vi "client.vi"() -> ()   [LabVIEW 2019]
uses:
  Generated_client/RPC Messages/Greeter_req.ctl
  Generated_client/RPC Messages/Greeter_req_req_oneof/Greeter_req_req_oneof.lvclass
  Generated_client/RPC Messages/Greeter_req_req_oneof/Greeter_req_req_oneof.lvclass/Greeter_req_req_oneof.ctl
  Generated_client/RPC Messages/Greeter_res_res_oneof/Greeter_res_res_oneof.lvclass/Greeter_res_res_oneof.ctl
  Generated_client/Generated_client.lvlib
  Generated_client/RPC Messages/Greeter_res_res_oneof/Greeter_res_res_oneof.lvclass
panel:
  out "res_price":sgl format="%.2f"
  out "res_flag":bool
  out "res_num":i32
  out "res_name":string
  out "res_latitude":i32
  in  "req_latitude":i32=1011
  in  "req_price":sgl=123.0
  in  "flag":bool
  in  "req_num":i32=12
  in  "req_name":string="Dan"
  in  "req_oneof":u16(ring) items=["req_name", "req_num", "flag", "price"]
  out "error out":errorcluster
  in  "error in":errorcluster
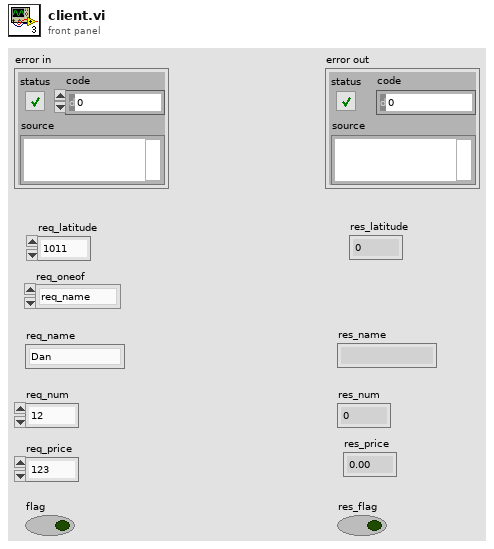
[diagram p1: front panel]
types:
  T1 = typedef "Generated_client.lvlib/Greeter_req.ctl" = cluster{"req_latitude":i32, "Greeter_req_req_oneof":refnum<class "Greeter_req_req_oneof.lvclass">}
  T2 = typedef "grpc-lvsupport-release.lvlib/grpcId.ctl" = u64
  T3 = typedef "Generated_client.lvlib/Greeter_res.ctl" = cluster{"res_latitude":i32, "Greeter_res_res_oneof":refnum<class "Greeter_res_res_oneof.lvclass">}
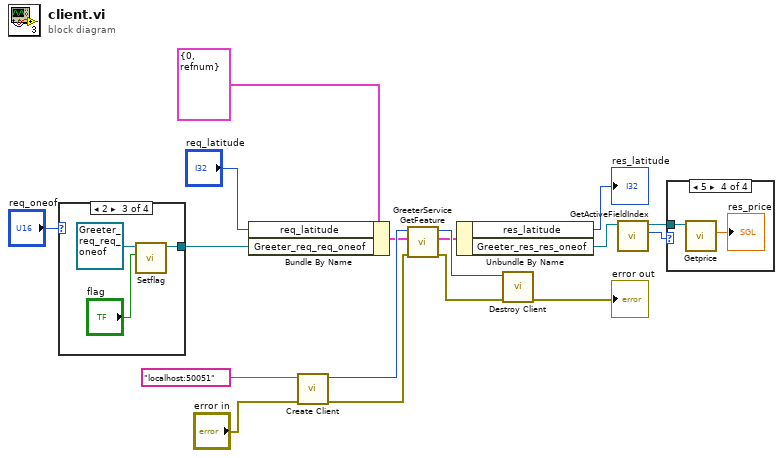
[diagram p0: block diagram]
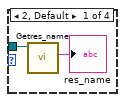
[diagram p2: hidden frame]
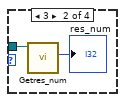
[diagram p3: hidden frame]
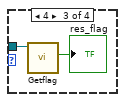
[diagram p4: hidden frame]
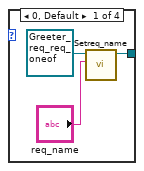
[diagram p5: hidden frame]
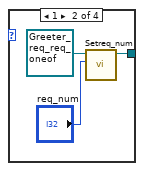
[diagram p6: hidden frame]
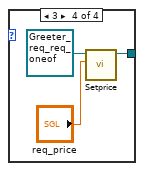
[diagram p7: hidden frame]
diagram:
  n1 = case shown="2" "req_oneof" {
    tunnel: [w18 w21 w26 w27] -> w7
    frame 0, Default {
      n2 = call "Setreq_name.vi"("Set_Val"="req_name", "OneOfTemplate in"=refnum<class "Greeter_req_req_oneof.lvclass"> refnum) -> ("OneOfTemplate out"=w18:refnum<class "Greeter_req_req_oneof.lvclass">)  [unwired: 8 in, 1 out]
    }
    frame 1 {
      n3 = call "Setreq_num.vi"("Set_Val"="req_num", "OneOfTemplate in"=refnum<class "Greeter_req_req_oneof.lvclass"> refnum) -> ("OneOfTemplate out"=w21:refnum<class "Greeter_req_req_oneof.lvclass">)  [unwired: 8 in, 1 out]
    }
    frame 2 {
      n4 = call "Setflag.vi"("Set_Val"="flag", "OneOfTemplate in"=refnum<class "Greeter_req_req_oneof.lvclass"> refnum) -> ("OneOfTemplate out"=w26:refnum<class "Greeter_req_req_oneof.lvclass">)  [unwired: 8 in, 1 out]
    }
    frame 3 {
      n5 = call "Setprice.vi"("Set_Val"="req_price", "OneOfTemplate in"=refnum<class "Greeter_req_req_oneof.lvclass"> refnum) -> ("OneOfTemplate out"=w27:refnum<class "Greeter_req_req_oneof.lvclass">)  [unwired: 8 in, 1 out]
    }
  }
  n6 = Bundle By Name(cluster=T1 {"req_latitude"=0, "Greeter_req_req_oneof"=refnum} ("Greeter_req"), "req_latitude"="req_latitude", "Greeter_req_req_oneof"=w7) -> (w6:T1)
  n7 = call "Create Client.vi"("error in"="error in", "address"="localhost:50051") -> ("error out"=w15:errorcluster, "gRPC ID Out"=w17:T2)  [unwired: 8 in]
  n8 = call "GreeterService GetFeature.vi"("error in"=w15, "Request Data"=w6, "gRPC ID"=w17) -> ("error out"=w14:errorcluster, "Response Data"=w5:T3, "gRPC ID out"=w16:T2)  [unwired: 6 in]
  n9 = Unbundle By Name(w5) -> ("res_latitude"=→"res_latitude":i32, "Greeter_res_res_oneof"=w3:refnum<class "Greeter_res_res_oneof.lvclass">)
  n10 = call "Destroy Client.vi"("error in"=w14, "gRPC ID"=w16) -> ("error out"=→"error out":errorcluster)  [unwired: 9 in]
  n11 = call "GetActiveFieldIndex.vi"("OneOfTemplate in"=w3) -> ("Active Field Index"=w2:i32, "OneOfTemplate out"=w1:refnum<class "Greeter_res_res_oneof.lvclass">)  [unwired: 8 in, 1 out]
  n12 = case shown="5" w2 {
    tunnel: w1 -> [w31 w33 w35 w37]
    frame 2, Default {
      n13 = call "Getres_name.vi"("OneOfTemplate in"=w31) -> ("Get_Val"=→"res_name":string)  [unwired: 8 in, 2 out]
    }
    frame 3 {
      n14 = call "Getres_num.vi"("OneOfTemplate in"=w33) -> ("Get_Val"=→"res_num":i32)  [unwired: 8 in, 2 out]
    }
    frame 4 {
      n15 = call "Getflag.vi"("OneOfTemplate in"=w35) -> ("Get_Val"=→"res_flag":bool)  [unwired: 8 in, 2 out]
    }
    frame 5 {
      n16 = call "Getprice.vi"("OneOfTemplate in"=w37) -> ("Get_Val"=→"res_price":sgl)  [unwired: 8 in, 2 out]
    }
  }
